vi "open.vi"(8 "error in (no error)":errorcluster, 11 "Function Generator in":refnum<class "Function Generator.lvclass">) -> (0 "error out":errorcluster, 3 "Function Generator out":refnum<class "Function Generator.lvclass">)   [LabVIEW 2020, in "Function Generator.lvclass"]
uses:
  Function Generator.lvclass
  Function Generator.lvclass/Function Generator.ctl
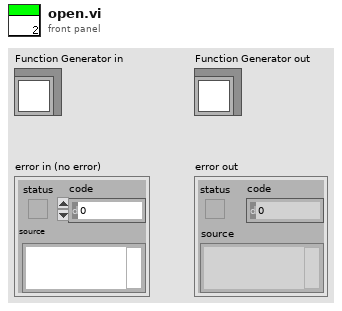
[diagram p1: front panel]
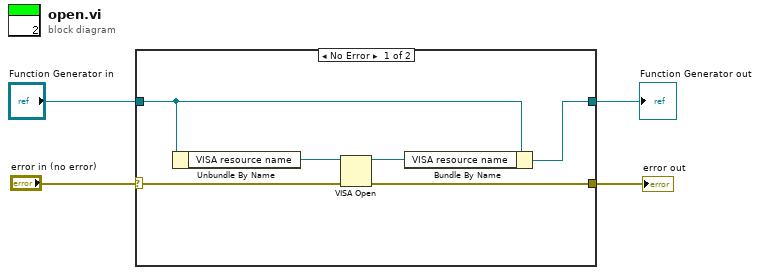
[diagram p0: block diagram]
diagram:
  n1 = case shown="No Error" "error in (no error)" {
    selector: "error in (no error)" -> [w5 w10]
    tunnel: "Function Generator in" -> [w9 w11]
    tunnel: [w8 w11] -> w2
    tunnel: [w5 w10] -> w1
    frame No Error {
      n2 = Unbundle By Name(w9) -> ("VISA resource name"=w7:refnum<visa-resource-name>)
      n3 = VISA Open(error in (no error)=w5, VISA resource name=w7) -> (VISA resource name=w6:refnum<visa-resource-name>)  [unwired: 3 in, 1 out]
      n4 = Bundle By Name(cluster=w9, "VISA resource name"=w6) -> (w8:refnum<class "Function Generator.lvclass">)
    }
    frame Error {
    }
  }
  "error out" <- w1
  "Function Generator out" <- w2
